vi "Handle Last Ack Core.vi"(4 "error in (no error)":errorcluster, 6 "Last Ack":refnum<class "Last Ack.lvclass">, 7 "Papa in":refnum<class "Papa.lvclass">) -> (0 "error out":errorcluster, 3 "Papa out":refnum<class "Papa.lvclass">)   [LabVIEW 2020, in "Papa.lvlib" / "Papa.lvclass"]
doc: "(<B>Filename</B>: Actor Framework.lvlib:Actor.lvclass:Handle Last Ack Core.vi)\n\nDefines how the caller actor responds to the Last Ack message from a nested actor. The Last Ack message is the final message a nested actor sends to its caller before it shuts down. The message contains information about the final state of the nested actor.\n\nBy default, this method does nothing except return any error the nested actor sent. A descendant class may override this method to define behavior."
uses:
  Papa.lvclass
  <vilib>/ActorFramework/LastAck/Last Ack.lvclass
  C:/Program Files (x86)/National Instruments/LabVIEW 2020/vi.lib/ActorFramework/Actor/Actor.lvclass
  Hijo/Hijo.lvclass
  <vilib>/ActorFramework/LastAck/Last Ack.lvclass/Last Ack.ctl
  Hijo/Hijo.lvclass/Hijo.ctl
  <vilib>/ActorFramework/Message Enqueuer/Message Enqueuer.lvclass
  Papa.lvclass/Papa.ctl
  <vilib>/ActorFramework/Actor/Actor.lvclass
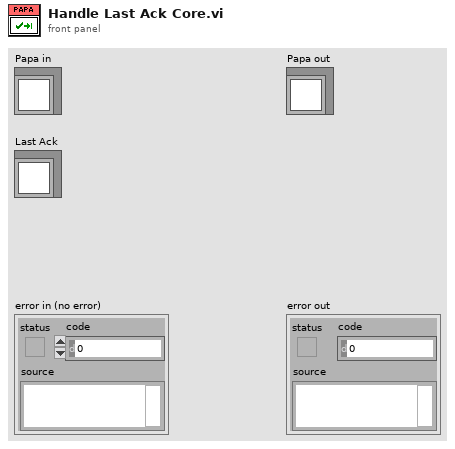
[diagram p1: front panel]
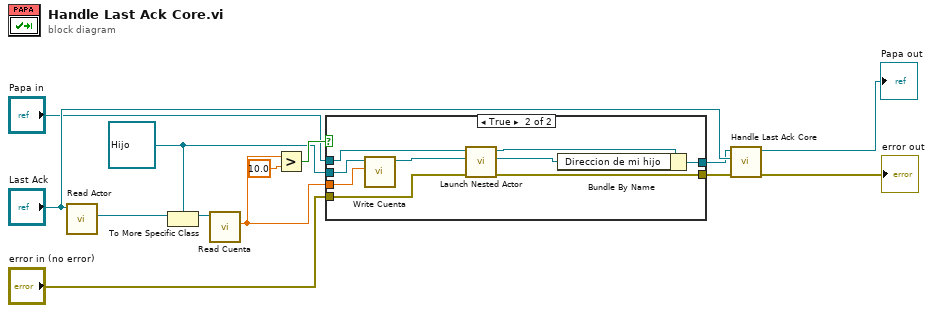
[diagram p0: block diagram]
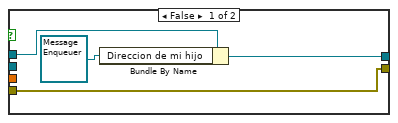
[diagram p2: hidden frame]
diagram:
  w8 = refnum<class "Hijo.lvclass"> refnum ("Hijo.lvlib:Hijo.lvclass")
  n1 = call <vilib>:"Read Actor.vi"("Last Ack"="Last Ack") -> ("Actor"=w12:refnum<class "Actor.lvclass">)  [unwired: 10 in]
  n2 = To More Specific Class(target class=w8, reference=w12) -> (specific class reference=w11:refnum<class "Hijo.lvclass">)  [unwired: 1 in, 1 out]
  n3 = call "Read Cuenta.vi"("Hijo in"=w11) -> ("Cuenta"=w7:dbl)  [unwired: 9 in, 1 out]
  n4 = Greater?(x=w7, y=10.0) -> (0:w9:bool)
  n5 = case shown="True" w9 {
    tunnel: [w14 w26] -> w4
    tunnel: "Papa in" -> [w17 w25]
    tunnel: w8 -> [_ w22]
    tunnel: w7 -> [_ w20]
    tunnel: [w15 w19] -> w5
    tunnel: "error in (no error)" -> [w14 w18]
    frame False {
      n6 = Bundle By Name(cluster=w17, "Direccion de mi hijo"=refnum<class "Message Enqueuer.lvclass"> refnum) -> (w15:refnum<class "Papa.lvclass">)
    }
    frame True {
      n7 = call "Write Cuenta.vi"("Cuenta"=w20, "Hijo in"=w22) -> ("Hijo out"=w21:refnum<class "Hijo.lvclass">)  [unwired: 9 in]
      n8 = call <vilib>:"Launch Nested Actor.vi"("error in (no error)"=w18, "Nested Actor"=w21, "Caller Actor in"=w25) -> ("error out"=w26:errorcluster, "Nested Actor's Enqueuer"=w23:refnum<class "Message Enqueuer.lvclass">, "Caller Actor out"=w24:refnum<class "Papa.lvclass">)  [unwired: 6 in]
      n9 = Bundle By Name(cluster=w24, "Direccion de mi hijo"=w23) -> (w19:refnum<class "Papa.lvclass">)
    }
  }
  n10 = call-parent "Handle Last Ack Core.vi"("error in (no error)"=w4, "Last Ack"="Last Ack", "Actor in"=w5) -> ("error out"=→"error out":errorcluster, "Actor out"=→"Papa out":refnum<class "Papa.lvclass">)  [unwired: 3 in]
